vi "move_motor.vi"(2 "error in (no error)":errorcluster caption="错误输入（无错误）", 3 "Basic Move Parameters":T1, 4 "StepMotor输入":refnum<class "StepMotor.lvclass">) -> (0 "error out":errorcluster caption="错误输出", 1 "StepMotor输出":refnum<class "StepMotor.lvclass">)   [LabVIEW 2016, in "MotionControl.lvlib" / "StepMotor.lvclass"]
uses:
  <userlib>/MotionControl/StepMotor/StepMotor.lvclass
  <userlib>/MotionControl/StepMotor/StepMotor.lvclass/StepMotor.ctl
  <userlib>/UISimCanFunc_wrapper/UISimCanFunc_wrapper.lvlib
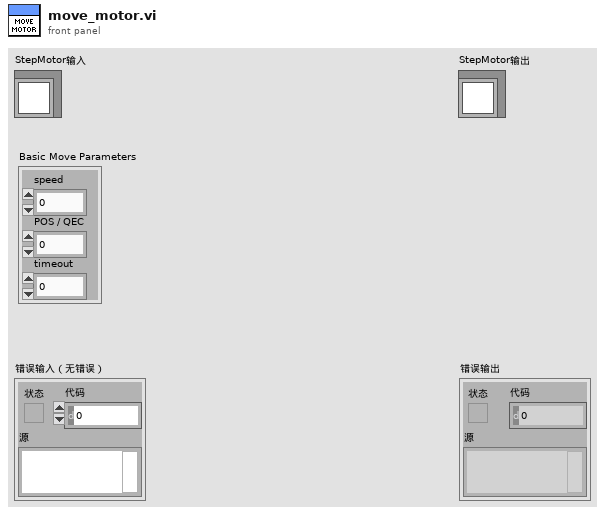
[diagram p1: front panel]
types:
  T1 = cluster{"speed":i32, "POS / QEC":i32, "timeout":i32}
  T2 = typedef "MotionControl.lvlib/StepMotor.lvclass/AdvMovePara.ctl" = cluster{"acceleration":i32, "deceleration":i32, "max startup speed":i32, "max stop speed":i32}
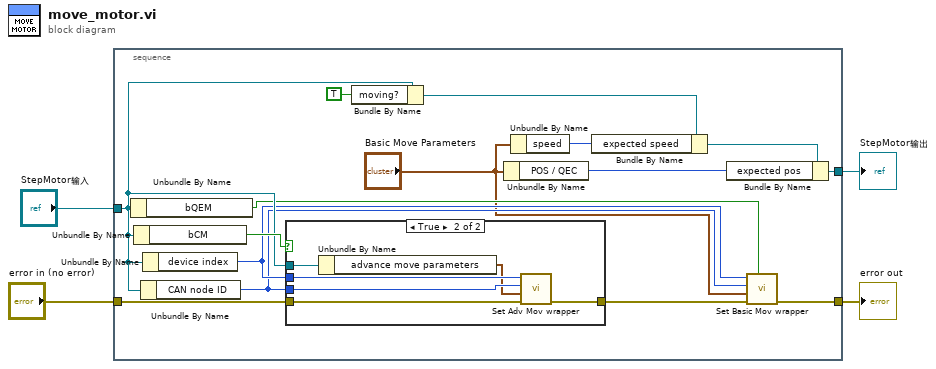
[diagram p0: block diagram]
diagram:
  n1 = stacked-sequence {
    tunnel: [w7] -> w4
    tunnel: [w16] -> w2
    tunnel: "StepMotor输入" -> [w13]
    tunnel: "error in (no error)" -> [w5]
    frame #0 {
      n2 = Unbundle By Name(w13) -> ("bQEM"=w12:bool)
      n3 = Unbundle By Name(w13) -> ("bCM"=w19:bool)
      n4 = Unbundle By Name(w13) -> ("CAN node ID"=w10:u32)
      n5 = Unbundle By Name(w13) -> ("device index"=w11:u32)
      n6 = case shown="True" w19 {
        tunnel: w11 -> [_ w25]
        tunnel: w10 -> [_ w24]
        tunnel: w5 -> [w20 w22]
        tunnel: [w20 w21] -> w8
        tunnel: w13 -> [_ w26]
        frame False {
        }
        frame True {
          n7 = Unbundle By Name(w26) -> ("advance move parameters"=w23:T2)
          n8 = call <userlib>:"Set Adv Mov wrapper.vi"("error in (no error)"=w22, "pAdvMovObj"=w23, "dwCanNodeId"=w24, "dwDevIndex"=w25) -> ("error out"=w21:errorcluster)  [unwired: 5 in, 2 out]
        }
      }
      n9 = Bundle By Name(cluster=w13, "moving?"=TRUE) -> (w18:refnum<class "StepMotor.lvclass">)
      n10 = Unbundle By Name("Basic Move Parameters") -> ("POS / QEC"=w14:i32)
      n11 = Unbundle By Name("Basic Move Parameters") -> ("speed"=w15:i32)
      n12 = Bundle By Name(cluster=w18, "expected speed"=w15) -> (w17:refnum<class "StepMotor.lvclass">)
      n13 = Bundle By Name(cluster=w17, "expected pos"=w14) -> (w16:refnum<class "StepMotor.lvclass">)
      n14 = call <userlib>:"Set Basic Mov wrapper.vi"("bLoop"=w12, "error in (no error)"=w8, "pBasicMovObj"="Basic Move Parameters", "dwCanNodeId"=w10, "dwDevIndex"=w11) -> ("error out"=w7:errorcluster)  [unwired: 4 in, 2 out]
    }
  }
  "error out" <- w4
  "StepMotor输出" <- w2
